vi "Scan To Text - Copy.vi"() -> ()   [LabVIEW 2022 SP3]
uses:
  <vilib>/userdefined/High Color/IMAQdx.ctl
  <vilib>/vision/driver/NI_Vision_Acquisition_Software.lvlib
  <vilib>/vision/NI_Vision_Development_Module.lvlib
panel:
  in  "Session In":T1
  in  "Rectangle":T2 {"Rotation" min=-90.0 max=90.0 step=1.0 format="%.2f"; "Left" scale=0.0..1024.0; "Right" scale=0.0..1024.0}
  in  "File Path":path
  out "Image 2":T3(plugin-control)
  out "Read String":string
  # "Project performed by"
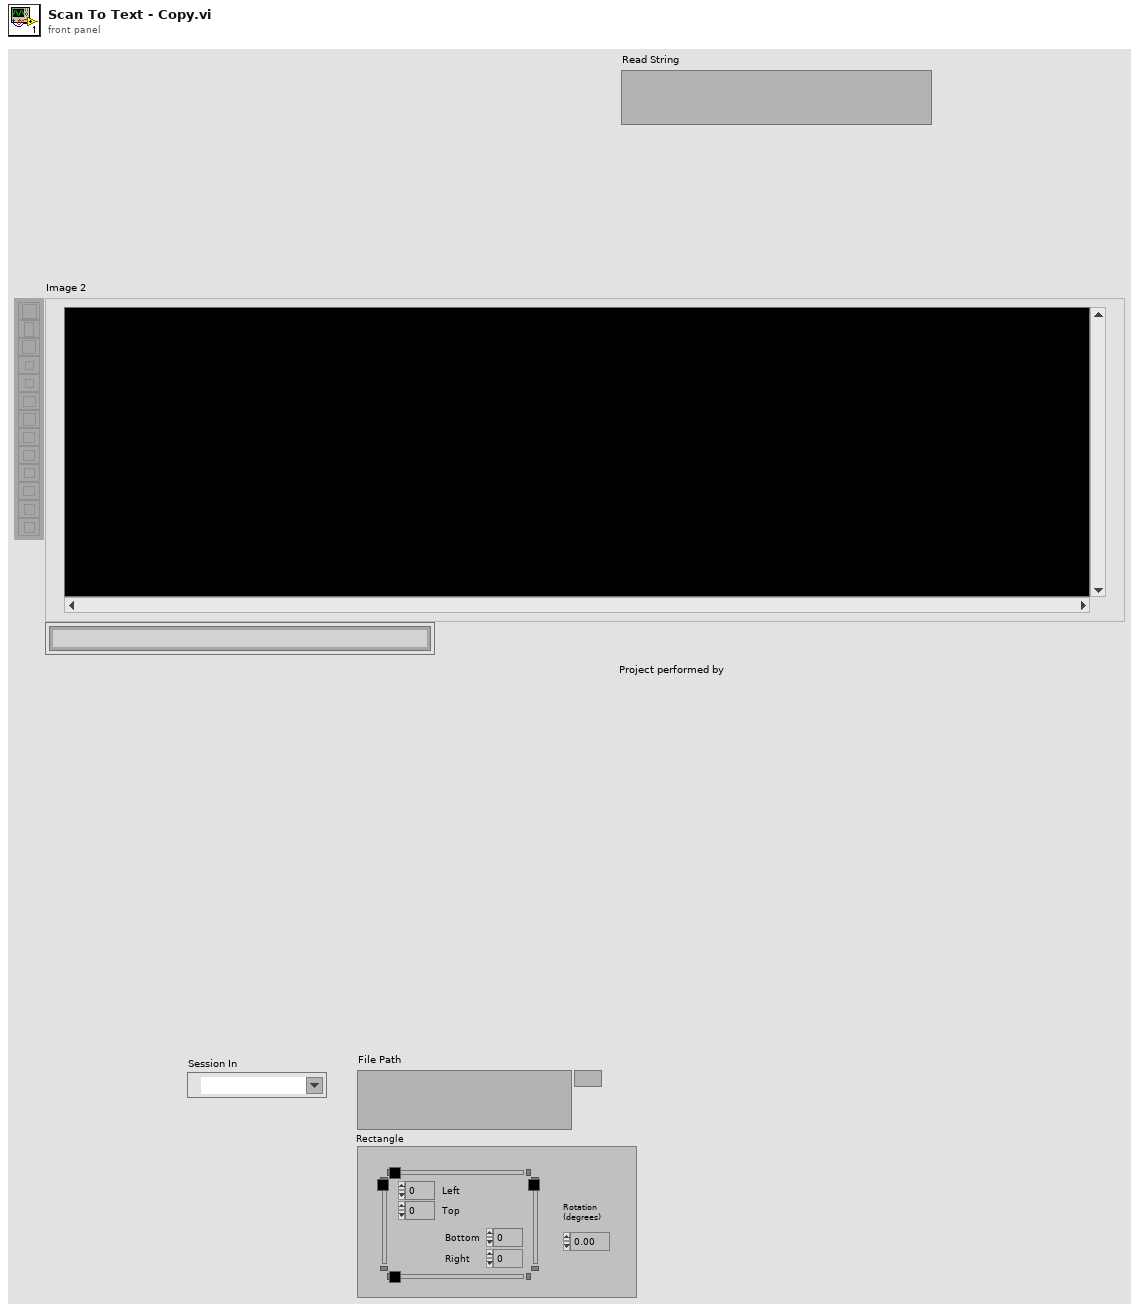
[diagram p1: front panel]
types:
  T1 = typedef "IMAQdx.ctl" = refnum<k21>
  T2 = typedef "IMAQ Rectangle" = cluster{"Left":i32, "Top":i32, "Right":i32, "Bottom":i32, "Rotation":dbl}
  T3 = typedef "IMAQ Image.ctl" = refnum<image>
  T4 = typedef "IMAQ OCR Session.ctl" = refnum<k1>
  T5 = typedef "ROI Descriptor" = cluster{"Global Rectangle":i32[], "Contours":cluster{"ID":enum32{"External", "Internal"}, "Type":u32, "Coordinates":i32[]}[]}
  T6 = cluster{"Global Rectangle":i32[], "Contours":cluster{"ID":enum32{"External", "Internal"}, "Type":u32, "Coordinates":i32[]}[]}
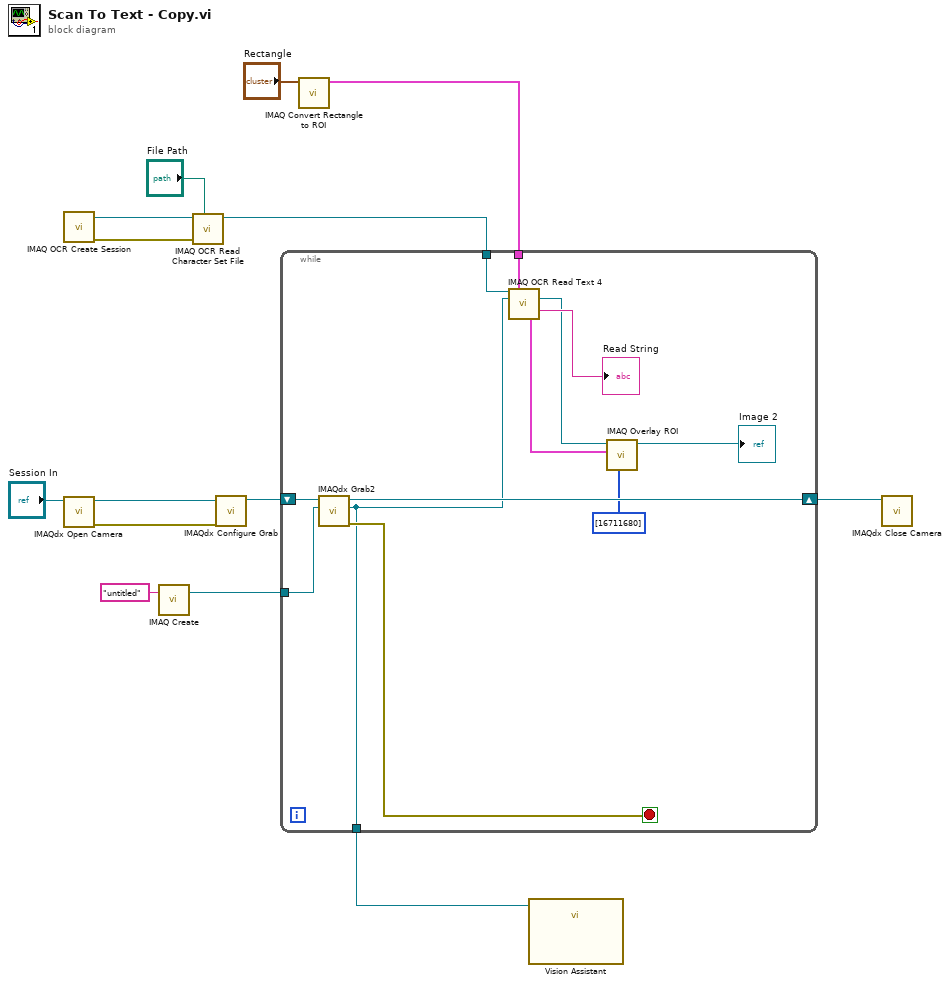
[diagram p0: block diagram]
diagram:
  n1 = call "IMAQ OCR Create Session"() -> ("error out"=w7:errorcluster, "IMAQ OCR Session"=w8:T4)  [unwired: 10 in]
  n2 = call <vilib>:"IMAQdx Open Camera.vi"("Session In"="Session In") -> ("error out"=w13:errorcluster, "Session Out"=w14:T1)  [unwired: 9 in]
  n3 = call "IMAQ Create"("Image Name"="untitled") -> ("New Image"=w10:T3)  [unwired: 4 in, 1 out]
  n4 = call "IMAQ OCR Read Character Set File"("File Path"="File Path", "error in (no error)"=w7, "IMAQ OCR Session"=w8) -> ("IMAQ OCR Session (dup)"=w6:T4)  [unwired: 6 in, 2 out]
  n5 = call <vilib>:"IMAQdx Configure Grab.vi"("error in"=w13, "Session In"=w14) -> ("Session Out"=w12:T1)  [unwired: 8 in, 1 out]
  n6 = call "IMAQ Convert Rectangle to ROI"("Rectangle"="Rectangle") -> ("ROI Descriptor"=w3:T5)  [unwired: 8 in, 1 out]
  n7 = while {
    shift-right: [w25] -> w11
    shift-left: w12 -> [w26]
    tunnel: w10 -> [w24]
    tunnel: w6 -> [w22]
    tunnel: w3 -> [w20]
    tunnel: [w15] -> w2
    stop <- w23 stop-if-true
    n8 = call <vilib>:"IMAQdx Grab2.vi"("Image In"=w24, "Session In"=w26) -> ("error out"=w23:errorcluster, "Image Out"=w15:T3, "Session Out"=w25:T1)  [unwired: 6 in, 1 out]
    n9 = call "IMAQ OCR Read Text 4"("IMAQ OCR Session"=w22, "ROI Descriptor"=w20, "Image"=w15) -> ("Image (dup)"=w18:T3, "Read String"=→"Read String":string, "ROI Bounding Characters"=w19:T6)  [unwired: 6 in, 4 out]
    n10 = call "IMAQ Overlay ROI"("Colors (Green)"=u32[] [16711680], "ROI Descriptor"=w19, "Image"=w18) -> ("Image Out"=→"Image 2":T3)  [unwired: 7 in, 1 out]
  }
  n11 = call "Vision Assistant"("Image In"=w2) -> ()  [unwired: 25 in, 2 out]
  n12 = call <vilib>:"IMAQdx Close Camera.vi"("Session In"=w11) -> ()  [unwired: 10 in, 1 out]
